vi "Czytaj_Plyta_Info.vi"(6 "Section":string, 7 "error in (no error)":errorcluster, 9 "key names":string[](array[string]), 10 "Refnum in":T1) -> (0 "error out":errorcluster, 3 "Refnum out":T1, 4 "Konfig Info":string[](array[string]))   [LabVIEW 2014]
uses:
  <vilib>/Utility/config.llb/Config Data RefNum.ctl
  <vilib>/Utility/config.llb/Read Key (String).vi
  <vilib>/Utility/config.llb/NI_LVConfig.lvlib
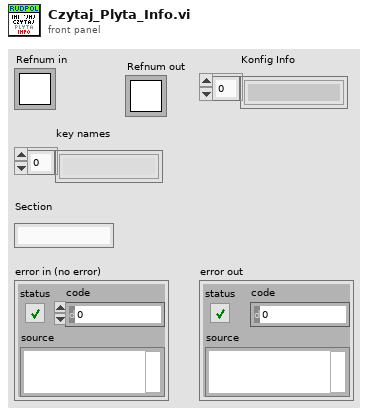
[diagram p1: front panel]
types:
  T1 = typedef "NI_LVConfig.lvlib/Config Data RefNum.ctl" = refnum<k1>
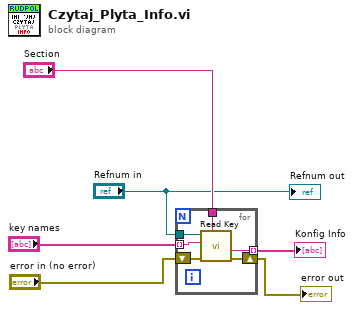
[diagram p0: block diagram]
diagram:
  n1 = for {
    shift-right: [w11] -> w3
    shift-left: "error in (no error)" -> [w12]
    tunnel: "Refnum in" -> [w10]
    tunnel: [w9] -> w4 mode=indexing
    tunnel: "key names" -> [w8] mode=indexing
    tunnel: "Section" -> [w7]
    n2 = call-poly <vilib>:"Read Key.vi"("section"=w7, "error in (no error)"=w12, "key"=w8, "refnum"=w10) -> ("error out"=w11:errorcluster, "value"=w9:string)  [unwired: 4 in, 2 out]
  }
  "Konfig Info" <- w4
  "error out" <- w3
  "Refnum out" <- "Refnum in"
